vi "Get Status Analog In.vi"(7 "error in (no error)":errorcluster, 9 "fReadData":i32, 10 "hdwf":i32) -> (0 "error out":errorcluster, 1 "psts":T1, 2 "function return":i32, 3 "hdwf out":i32)   [LabVIEW 2012, in "AnalogDiscSDKLv.lvlib"]
doc: "extern \"C\" __declspec(dllexport) int GetStatus_AnalogIn(HDWF hdwf,\n int fReadData,\n STS* psts\n );"
uses:
  <instrlib>/AnalogDiscSDKLv/AnalogDiscSDKLv.lvlib
  <instrlib>/AnalogDiscSDKLv/VIs/DWF_InstrumentStatus.ctl
  <instrlib>/AnalogDiscSDKLv/AnalogDiscSDKLv.dll
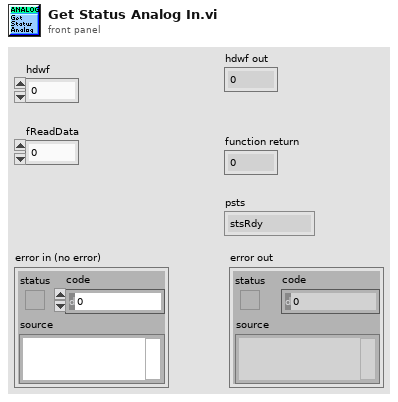
[diagram p1: front panel]
types:
  T1 = typedef "DWF_InstrumentStatus.ctl" = enum16{"stsRdy", "stsARM", "stsDone", "stsTrig", "stsCfg", "stsPrefill", "stsNotDone", "stsTrigDly", "stsError", "stsBusy", "stsStop"}
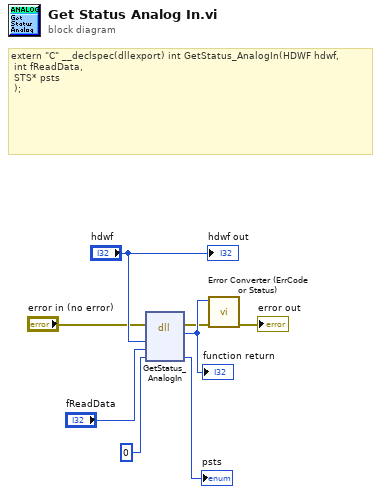
[diagram p0: block diagram]
diagram:
  # "extern \"C\" __declspec(dllexport) int GetStatus_AnalogIn(HDWF hdwf,\n\tint fReadData,\n\tSTS* psts\n\t);"
  n1 = dll-call lib="C:/Program Files (x86)/National Instruments/LabVIEW 2012/instr.lib/AnalogDiscSDKLv/AnalogDiscSDKLv.*" fn="GetStatus_AnalogIn"(error in="error in (no error)", "hdwf"="hdwf", "fReadData"="fReadData", "psts"=u8 0) -> (error out=w4:errorcluster, "return type"=w8:i32, "psts"=→"psts":u8)  [unwired: 4 in, 1 out]
  "function return" <- w8
  n2 = call <instrlib>:"Error Converter (ErrCode or Status).vi"("error in (no error)"=w4, "error code"=w8) -> ("error out"=→"error out":errorcluster)  [unwired: 9 in]
  "hdwf out" <- "hdwf"
